vi "pARCIAL-MILLER.vi"() -> ()   [LabVIEW 2017]
uses:
  miller/vis_variables.vi
  miller/Actuadores.vi
  miller/Alarmas.vi
  miller/Temperaturas.vi
  miller/Animaciones.vi
  miller/Pos_def.vi
  miller/Panela_R.vi
  miller/Cuadrada.vi
  miller/Pos_Modf.vi
panel:
  out "Molde Cuadrado":bool
  out "ALARMA TEMPERATURA FUERA DE\nNORMA":bool
  out "Temperatura Enfriador":dbl
  out "ALARMA DE  BAJA TEMPERATURA":bool
  out "ALARMA DE  ALTA TEMPERATURA":bool
  out "Temperatura Calentador":dbl
  out "Valvula\n Filtrado":bool
  out "ALARMA DE LLENADO":bool
  out "SENSOR DE CAÑA":bool
  out "Valvula\nCalentador":bool
  out "panela_liquida":bool
  out "guarapo":bool
  out "PANELA-R":bool
  out "Molde Redondo":bool
  out "bagazo":bool
  out "trituradora":bool
  out "caña":bool
  in  "Panela Cuadrada":bool
  in  "Panela Redonda":bool
  out "caja":bool
  out "PANELA-C":bool
  out "Carro_caña":bool
  out "carro_vaciando":bool
  out "Porcion de Caña":bool
  # "TRANZPORTAR"
  # "TRITURARADORA"
  # "TRITURAR"
  # "FILTRADO"
  # "FILTRAR"
  # "ENFRIADOR"
  # "CALENTADOR"
  # "CALENTAR"
  # "ZELECCION DE PANELA"
  # "ENFRIAR"
  # "EMPACAR"
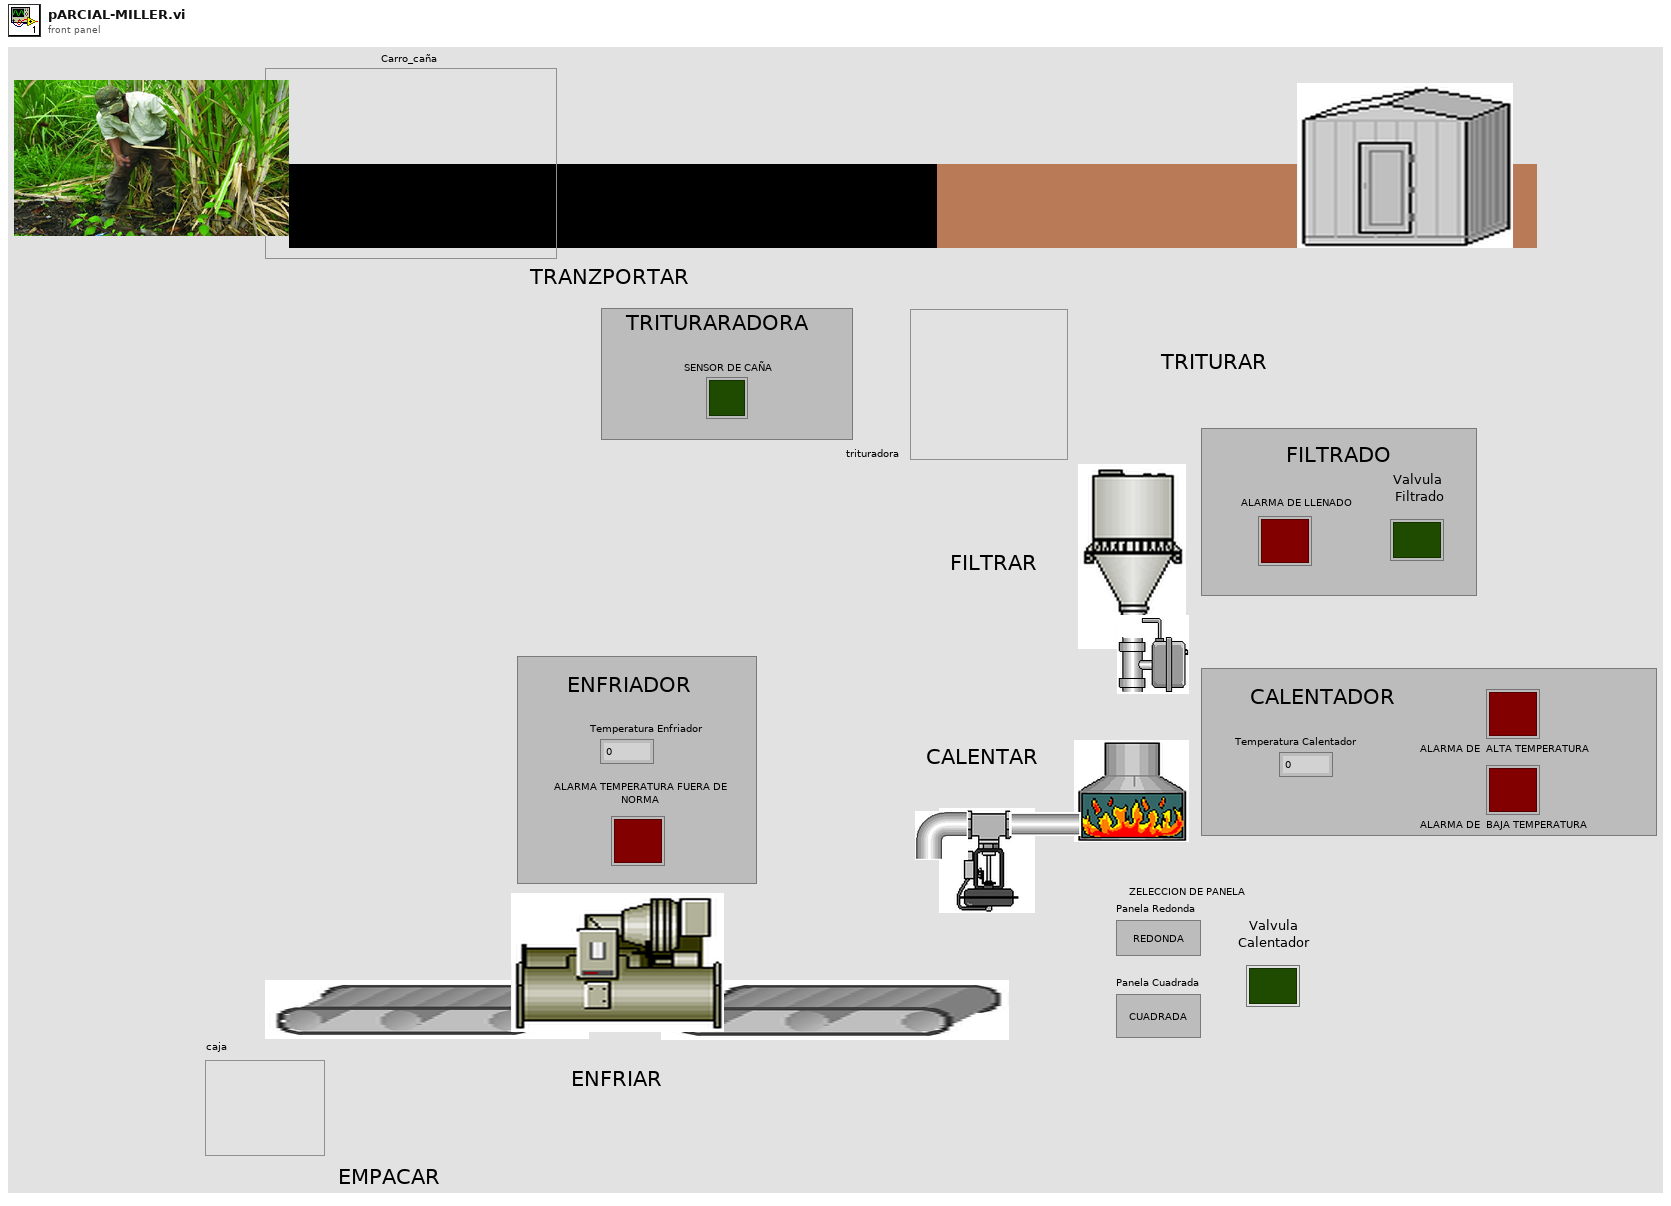
[diagram p1: front panel]
types:
  T1 = cluster{"Pos Carro Caña":i32, "Pos Porcion Caña ":i32, "Pos Moldes_R":i32, "Pos Panelas_R":i32, "Pos Panelas_C":i32, "Pos Moldes _C":i32}
  T2 = cluster{"Temperatura Calentador":dbl, "Temperatura Enfriador":dbl}
  T3 = cluster{"A_llenado":bool, "A_T_Fuera_Norma":bool, "A_Alta_temperatura":bool, "A_Baja_temperatura ":bool}
  T4 = cluster{"Valvula Filtrado":bool, "Valvula Calentador":bool}
  T5 = cluster{"vis carro caña":bool, "vis carro  vaciando":bool, "vis caña":bool, "vis porcion de caña":bool, "vis bagazo":bool, "vis guarapo":bool, " vis panela liquida":bool, " vis molde redondo":bool, " vis molde cuadrado":bool}
  T6 = cluster{"Pos_Modf_Carro_Caña":i32, "Pos_Modf_Porcion_Caña":i32, "Pos_Modf_Molde_Redondo":i32, "Pos_Modf_Molde_Cuadrado":i32, "Pos_Modf_Panela_R":i32, "Pos_Modf_Panela_C":i32}
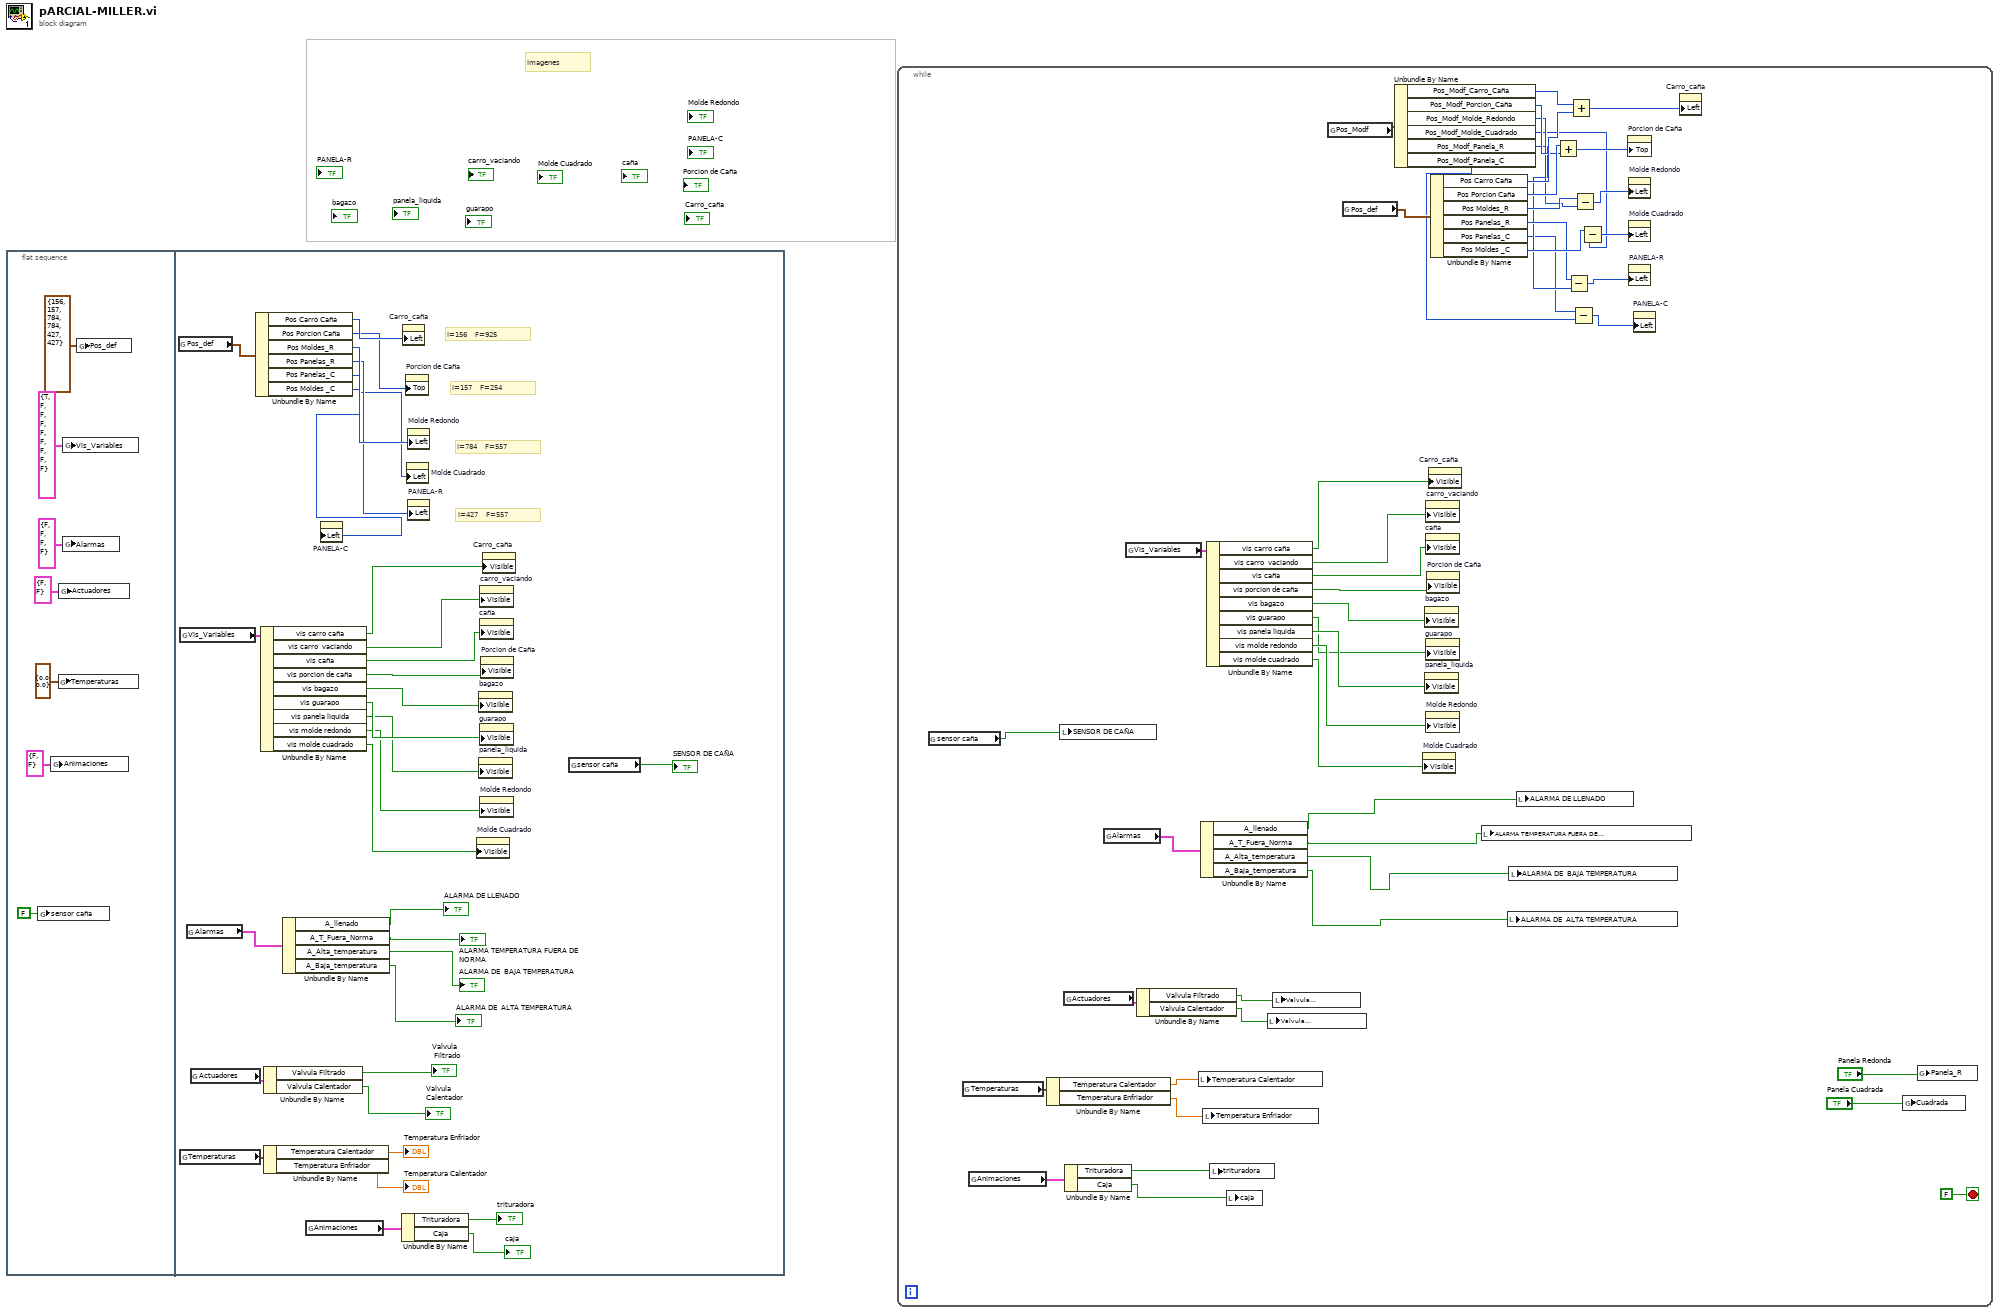
[diagram p0: block diagram]
diagram:
  # "Imagenes"
  n1 = flat-sequence {
    frame #0 {
      n2 = global write "senor caña.vi" "sensor caña"(FALSE ("sensor caña")) -> ()
      n3 = global write "Animaciones.vi" "Animaciones"(cluster{"Trituradora":bool, " Caja":bool} {"Trituradora"=FALSE, " Caja"=FALSE} ("Animaciones")) -> ()
      n4 = global write "Temperaturas.vi" "Temperaturas"(T2 {"Temperatura Calentador"=0.0, "Temperatura Enfriador"=0.0} ("Temperaturas")) -> ()
      n5 = global write "Actuadores.vi" "Actuadores"(T4 {"Valvula Filtrado"=FALSE, "Valvula Calentador"=FALSE} ("Actuadores")) -> ()
      n6 = global write "vis_variables.vi" "Vis_Variables"(T5 {"vis carro caña"=TRUE, "vis carro  vaciando"=FALSE, "vis caña"=FALSE, "vis porcion de caña"=FALSE, "vis bagazo"=FALSE, "vis guarapo"=FALSE, " vis panela liquida"=FALSE, " vis molde redondo"=FALSE, " vis molde cuadrado"=FALSE} ("Vis_Variables")) -> ()
      n7 = global write "Alarmas.vi" "Alarmas"(T3 {"A_llenado"=FALSE, "A_T_Fuera_Norma"=FALSE, "A_Alta_temperatura"=FALSE, "A_Baja_temperatura "=FALSE} ("Alarmas")) -> ()
      n8 = global write "Pos_def.vi" "Pos_def"(T1 {"Pos Carro Caña"=156, "Pos Porcion Caña "=157, "Pos Moldes_R"=784, "Pos Panelas_R"=784, "Pos Panelas_C"=427, "Pos Moldes _C"=427} ("Pos_def")) -> ()
    }
    frame #1 {
      # "I=427    F=557"
      # "I=784    F=557"
      # "I=157    F=254"
      # "I=156    F=925"
      n9 = global read "Pos_def.vi" "Pos_def"() -> (w15:T1)
      n10 = global read "vis_variables.vi" "Vis_Variables"() -> (w39:T5)
      n11 = global read "Temperaturas.vi" "Temperaturas"() -> (w21:T2)
      n12 = global read "Alarmas.vi" "Alarmas"() -> (w29:T3)
      n13 = global read "Actuadores.vi" "Actuadores"() -> (w26:T4)
      n14 = Unbundle By Name(w15) -> ("Pos Carro Caña"=w14:i32, "Pos Porcion Caña"=w13:i32, "Pos Moldes_R"=w12:i32, "Pos Panelas_R"=w11:i32, "Pos Panelas_C"=w10:i32, "Pos Moldes _C"=w9:i32)
      n15 = Unbundle By Name(w39) -> ("vis carro caña"=w38:bool, "vis carro  vaciando"=w37:bool, "vis caña"=w36:bool, "vis porcion de caña"=w35:bool, "vis bagazo"=w34:bool, "vis guarapo"=w33:bool, "vis panela liquida"=w32:bool, "vis molde redondo"=w31:bool, "vis molde cuadrado"=w30:bool)
      n16 = Unbundle By Name(w26) -> ("Valvula Filtrado"=→"Valvula\n Filtrado":bool, "Valvula Calentador"=→"Valvula\nCalentador":bool)
      n17 = Unbundle By Name(w21) -> ("Temperatura Calentador"=→"Temperatura Enfriador":dbl, "Temperatura Enfriador"=→"Temperatura Calentador":dbl)
      n18 = Unbundle By Name(w29) -> ("A_llenado"=→"ALARMA DE LLENADO":bool, "A_T_Fuera_Norma"=→"ALARMA TEMPERATURA FUERA DE\nNORMA":bool, "A_Alta_temperatura"=→"ALARMA DE  BAJA TEMPERATURA":bool, "A_Baja_temperatura"=→"ALARMA DE  ALTA TEMPERATURA":bool)
      n19 = global read "Animaciones.vi" "Animaciones"() -> (w18:cluster{"Trituradora":bool, " Caja":bool})
      n20 = property on="PANELA-C" class="Bool (strict)"("Left"=w10) -> ()  [unwired: 2 in, 2 out]
      n21 = Unbundle By Name(w18) -> ("Trituradora"=→"trituradora":bool, "Caja"=→"caja":bool)
      n22 = property on="Carro_caña" class="Bool (strict)"("Left"=w14) -> ()  [unwired: 2 in, 2 out]
      n23 = property on="Porcion de Caña" class="Bool (strict)"("Top"=w13) -> ()  [unwired: 2 in, 2 out]
      n24 = property on="Molde Cuadrado" class="Bool (strict)"("Left"=w9) -> ()  [unwired: 2 in, 2 out]
      n25 = property on="Molde Redondo" class="Bool (strict)"("Left"=w12) -> ()  [unwired: 2 in, 2 out]
      n26 = property on="PANELA-R" class="Bool (strict)"("Left"=w11) -> ()  [unwired: 2 in, 2 out]
      n27 = property on="Molde Cuadrado" class="Bool (strict)"("Visible"=w30) -> ()  [unwired: 2 in, 2 out]
      n28 = property on="bagazo" class="Bool (strict)"("Visible"=w34) -> ()  [unwired: 2 in, 2 out]
      n29 = property on="panela_liquida" class="Bool (strict)"("Visible"=w32) -> ()  [unwired: 2 in, 2 out]
      n30 = property on="carro_vaciando" class="Bool (strict)"("Visible"=w37) -> ()  [unwired: 2 in, 2 out]
      n31 = property on="caña" class="Bool (strict)"("Visible"=w36) -> ()  [unwired: 2 in, 2 out]
      n32 = property on="guarapo" class="Bool (strict)"("Visible"=w33) -> ()  [unwired: 2 in, 2 out]
      n33 = property on="Molde Redondo" class="Bool (strict)"("Visible"=w31) -> ()  [unwired: 2 in, 2 out]
      n34 = property on="Porcion de Caña" class="Bool (strict)"("Visible"=w35) -> ()  [unwired: 2 in, 2 out]
      n35 = property on="Carro_caña" class="Bool (strict)"("Visible"=w38) -> ()  [unwired: 2 in, 2 out]
      n36 = global read "senor caña.vi" "sensor caña"() -> (→"SENSOR DE CAÑA":bool)
    }
  }
  n37 = while {
    stop <- FALSE stop-if-true
    n38 = global read "senor caña.vi" "sensor caña"() -> (w40:bool)
    n39 = global read "Temperaturas.vi" "Temperaturas"() -> (w52:T2)
    n40 = global read "Animaciones.vi" "Animaciones"() -> (w51:cluster{"Trituradora":bool, " Caja":bool})
    n41 = Unbundle By Name(w52) -> ("Temperatura Calentador"=w48:dbl, "Temperatura Enfriador"=w47:dbl)
    n42 = local write "SENSOR DE CAÑA"(w40) -> ()
    n43 = global read "Actuadores.vi" "Actuadores"() -> (w53:T4)
    n44 = Unbundle By Name(w51) -> ("Trituradora"=w50:bool, "Caja"=w49:bool)
    n45 = global read "Alarmas.vi" "Alarmas"() -> (w54:T3)
    n46 = global read "vis_variables.vi" "Vis_Variables"() -> (w55:T5)
    n47 = Unbundle By Name(w53) -> ("Valvula Filtrado"=w46:bool, "Valvula Calentador"=w45:bool)
    n48 = local write "Temperatura Calentador"(w48) -> ()
    n49 = Unbundle By Name(w54) -> ("A_llenado"=w44:bool, "A_T_Fuera_Norma"=w43:bool, "A_Alta_temperatura"=w42:bool, "A_Baja_temperatura"=w41:bool)
    n50 = local write "Temperatura Enfriador"(w47) -> ()
    n51 = Unbundle By Name(w55) -> ("vis carro caña"=w56:bool, "vis carro  vaciando"=w57:bool, "vis caña"=w58:bool, "vis porcion de caña"=w59:bool, "vis bagazo"=w60:bool, "vis guarapo"=w61:bool, "vis panela liquida"=w62:bool, "vis molde redondo"=w63:bool, "vis molde cuadrado"=w64:bool)
    n52 = local write "trituradora"(w50) -> ()
    n53 = local write "caja"(w49) -> ()
    n54 = local write "Valvula\nCalentador"(w45) -> ()
    n55 = local write "Valvula\n Filtrado"(w46) -> ()
    n56 = global read "Pos_Modf.vi" "Pos_Modf"() -> (w85:T6)
    n57 = global read "Pos_def.vi" "Pos_def"() -> (w86:T1)
    n58 = Unbundle By Name(w85) -> ("Pos_Modf_Carro_Caña"=w82:i32, "Pos_Modf_Porcion_Caña"=w79:i32, "Pos_Modf_Molde_Redondo"=w77:i32, "Pos_Modf_Molde_Cuadrado"=w73:i32, "Pos_Modf_Panela_R"=w71:i32, "Pos_Modf_Panela_C"=w68:i32)
    n59 = property on="Molde Cuadrado" class="Bool (strict)"("Visible"=w64) -> ()  [unwired: 2 in, 2 out]
    n60 = property on="bagazo" class="Bool (strict)"("Visible"=w60) -> ()  [unwired: 2 in, 2 out]
    n61 = property on="panela_liquida" class="Bool (strict)"("Visible"=w62) -> ()  [unwired: 2 in, 2 out]
    n62 = property on="carro_vaciando" class="Bool (strict)"("Visible"=w57) -> ()  [unwired: 2 in, 2 out]
    n63 = property on="caña" class="Bool (strict)"("Visible"=w58) -> ()  [unwired: 2 in, 2 out]
    n64 = property on="guarapo" class="Bool (strict)"("Visible"=w61) -> ()  [unwired: 2 in, 2 out]
    n65 = property on="Molde Redondo" class="Bool (strict)"("Visible"=w63) -> ()  [unwired: 2 in, 2 out]
    n66 = property on="Porcion de Caña" class="Bool (strict)"("Visible"=w59) -> ()  [unwired: 2 in, 2 out]
    n67 = property on="Carro_caña" class="Bool (strict)"("Visible"=w56) -> ()  [unwired: 2 in, 2 out]
    n68 = Unbundle By Name(w86) -> ("Pos Carro Caña"=w83:i32, "Pos Porcion Caña"=w80:i32, "Pos Moldes_R"=w78:i32, "Pos Panelas_R"=w72:i32, "Pos Panelas_C"=w69:i32, "Pos Moldes _C"=w74:i32)
    n69 = local write "ALARMA TEMPERATURA FUERA DE\nNORMA"(w43) -> ()
    n70 = local write "ALARMA DE  ALTA TEMPERATURA"(w41) -> ()
    n71 = local write "ALARMA DE  BAJA TEMPERATURA"(w42) -> ()
    n72 = local write "ALARMA DE LLENADO"(w44) -> ()
    n73 = Add(x=w80, y=w79) -> (x+y=w81:i32)
    n74 = Subtract(x=w72, y=w71) -> (x-y=w70:i32)
    n75 = Add(x=w82, y=w83) -> (x+y=w84:i32)
    n76 = Subtract(x=w69, y=w68) -> (x-y=w67:i32)
    n77 = Subtract(x=w78, y=w77) -> (x-y=w76:i32)
    n78 = Subtract(x=w74, y=w73) -> (x-y=w75:i32)
    n79 = property on="Porcion de Caña" class="Bool (strict)"("Top"=w81) -> ()  [unwired: 2 in, 2 out]
    n80 = property on="Molde Redondo" class="Bool (strict)"("Left"=w76) -> ()  [unwired: 2 in, 2 out]
    n81 = property on="Molde Cuadrado" class="Bool (strict)"("Left"=w75) -> ()  [unwired: 2 in, 2 out]
    n82 = property on="PANELA-R" class="Bool (strict)"("Left"=w70) -> ()  [unwired: 2 in, 2 out]
    n83 = property on="PANELA-C" class="Bool (strict)"("Left"=w67) -> ()  [unwired: 2 in, 2 out]
    n84 = property on="Carro_caña" class="Bool (strict)"("Left"=w84) -> ()  [unwired: 2 in, 2 out]
    n85 = global write "Cuadrada.vi" "Cuadrada"("Panela Cuadrada") -> ()
    n86 = global write "Panela_R.vi" "Panela_R"("Panela Redonda") -> ()
  }
